vi "RpeakDetector.vi"() -> ()   [LabVIEW 2026]
uses:
  <vilib>/Waveform/WDTOps.llb/WDT Waveform to XY Pairs DBL.vi
  <vilib>/Analysis/NI_AAL_SigProc.lvlib
panel:
  out "Waveform Graph":waveform(dbl)[](graph)
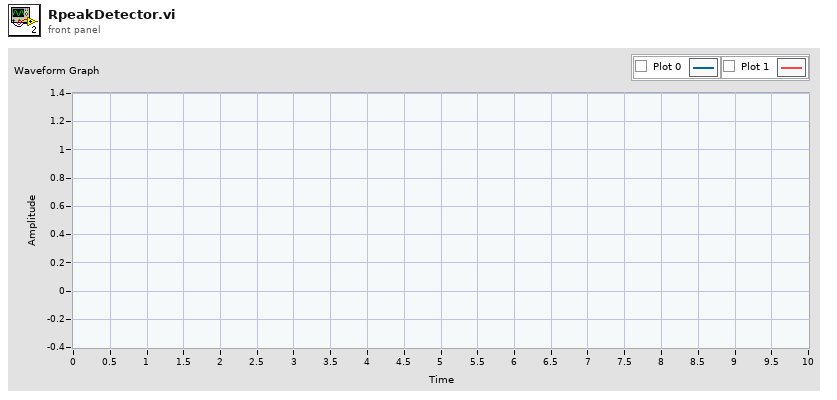
[diagram p1: front panel]
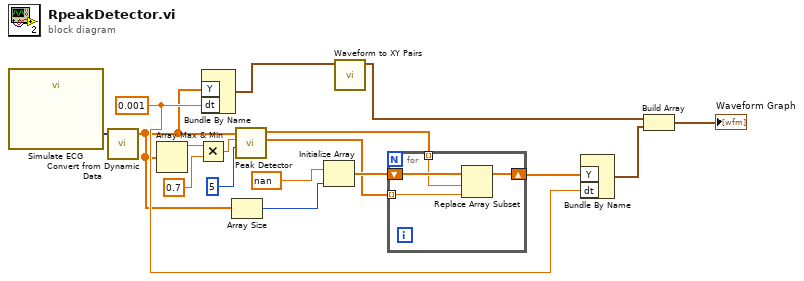
[diagram p0: block diagram]
diagram:
  w6 = 0.001 ("dt")
  n1 = call "Simulate ECG"() -> ("ECG"=w17:dynamicdata)  [unwired: 10 in, 1 out]
  n2 = call "Convert from Dynamic Data"("Dynamic Data Type"=w17) -> ("Array"=w4:dbl[])  [unwired: 3 in]
  n3 = Array Max & Min(array=w4) -> (max value=w3:dbl)  [unwired: 3 out]
  n4 = Multiply(x=w3, y=0.7) -> (x*y=w1:dbl)
  n5 = Bundle By Name("Y"=w4, "dt"=w6) -> (w15:waveform(dbl))  [unwired: 1 in]
  n6 = Array Size(array=w4) -> (size(s)=w13:i32)
  n7 = call <vilib>:"Peak Detector.vi"("width"=5, "threshold"=w1, "X"=w4) -> ("Amplitudes"=w9:dbl[], "Locations"=w10:dbl[])  [unwired: 4 in, 3 out]
  n8 = Initialize Array(nan, w13) -> (w11:dbl[])
  n9 = call-poly <vilib>:"Waveform to XY Pairs.vi"("waveform in"=w15) -> ("waveform out"=w14:waveform(dbl))  [unwired: 8 in, 2 out]
  n10 = for {
    tunnel: w10 -> [w20] mode=indexing
    tunnel: w9 -> [w19] mode=indexing
    shift-right: [w18] -> w7
    shift-left: w11 -> [w21]
    n11 = Replace Array Subset(array=w21, new element=w19, index=w20) -> (w18:dbl[])
  }
  n12 = Bundle By Name("Y"=w7, "dt"=w6) -> (w5:waveform(dbl))  [unwired: 1 in]
  n13 = Build Array(w14, w5) -> (→"Waveform Graph":waveform(dbl)[])
